vi "Read Height.vi"(8 "error in (no error)":errorcluster, 11 "Solution Triangle in":refnum<class "Solution Triangle.lvclass">) -> (0 "error out":errorcluster, 2 "height":dbl, 3 "Solution Triangle out":refnum<class "Solution Triangle.lvclass">)   [LabVIEW 2015, in "Solution Triangle.lvclass"]
uses:
  Solution Triangle.lvclass
  Solution Triangle.lvclass/Solution Triangle.ctl
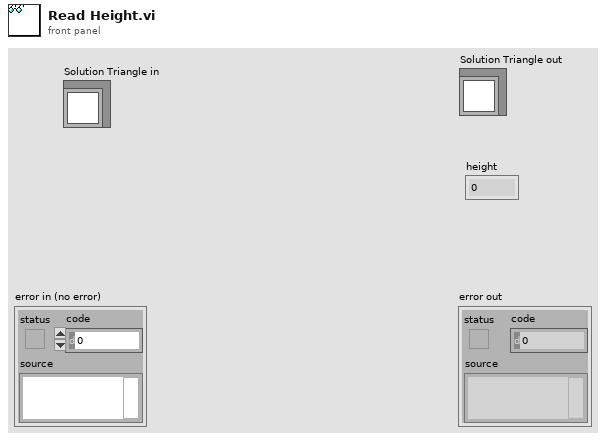
[diagram p1: front panel]
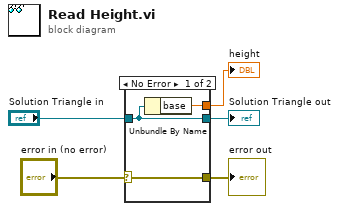
[diagram p0: block diagram]
diagram:
  n1 = case shown="No Error" "error in (no error)" {
    selector: "error in (no error)" -> [w8 w9]
    tunnel: [w8 w9] -> w4
    tunnel: [w7 w10] -> w1
    tunnel: "Solution Triangle in" -> [w7 w10]
    tunnel: [w6 _] -> w2
    frame No Error {
      n2 = Unbundle By Name(w7) -> ("base"=w6:dbl)
    }
    frame Error {
    }
  }
  "error out" <- w4
  "height" <- w2
  "Solution Triangle out" <- w1
